vi "故障数值解析.vi"(3 "输入":u8 format="%x") -> (0 "结果":string[](array[string]), 1 "颜色":u32[](array[colorbox]))   [LabVIEW 2013]
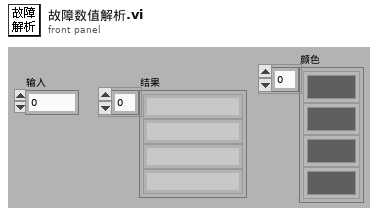
[diagram p1: front panel]
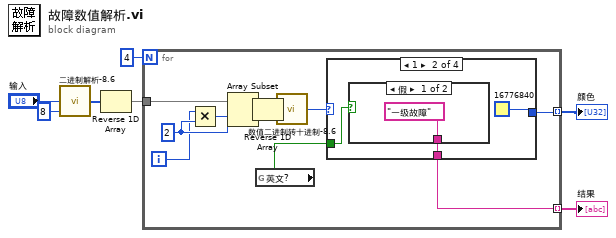
[diagram p0: block diagram]
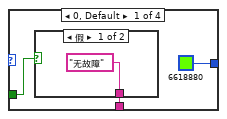
[diagram p2: hidden frame]
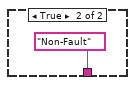
[diagram p3: hidden frame]
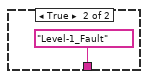
[diagram p4: hidden frame]
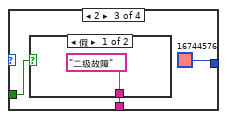
[diagram p5: hidden frame]
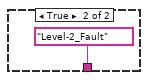
[diagram p6: hidden frame]
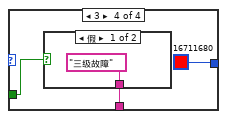
[diagram p7: hidden frame]
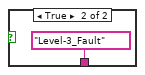
[diagram p8: hidden frame]
diagram:
  n1 = call "二进制解析-8.6.vi"("索引"=8, "数值"="输入") -> ("低位子数组"=w7:i32[])  [unwired: 1 in, 2 out]
  n2 = Reverse 1D Array(array=w7) -> (reversed array=w5:i32[])
  n3 = for {
    N: 4 -> [_]
    tunnel: w5 -> [w17]
    tunnel: [w8] -> w2 mode=indexing
    tunnel: [w11] -> w4 mode=indexing
    i -> [w12]
    w15 = 2
    n4 = Multiply(x=w12, y=w15) -> (x*y=w16:i32)
    n5 = Array Subset(array=w17, index=w16, length=w15) -> (w14:i32[])
    n6 = Reverse 1D Array(array=w14) -> (reversed array=w10:i32[])
    n7 = global read "中英文全局-8.6.vi" "英文?"() -> (w9:bool)
    n8 = call "数值二进制转十进制-8.6.vi"("子数组"=w10) -> ("十进制数值"=w13:i32)  [unwired: 4 out]
    n9 = case shown="1" w13 {
      tunnel: [w20 w25 w30 w35] -> w8
      tunnel: [u32 6618880 u32 16776840 u32 16744576 u32 16711680] -> w11
      tunnel: w9 -> [w18 w23 w28 w33]
      frame 0, Default {
        n10 = case shown="假" w18 {
          tunnel: ["无故障" "Non-Fault"] -> w20
          frame False {
          }
          frame True {
          }
        }
      }
      frame 1 {
        n11 = case shown="假" w23 {
          tunnel: ["一级故障" "Level-1_Fault"] -> w25
          frame False {
          }
          frame True {
          }
        }
      }
      frame 2 {
        n12 = case shown="假" w28 {
          tunnel: ["二级故障" "Level-2_Fault"] -> w30
          frame False {
          }
          frame True {
          }
        }
      }
      frame 3 {
        n13 = case shown="假" w33 {
          tunnel: ["三级故障" "Level-3_Fault"] -> w35
          frame False {
          }
          frame True {
          }
        }
      }
    }
  }
  "颜色" <- w4
  "结果" <- w2
